vi "IPS120_status.vi"(0 "Address":T1, 1 "error in":errorcluster) -> (2 "Set point":string, 3 "Real Field":string, 4 "Staus":string, 5 "Magnet Failed?":bool, 6 "Arrive":bool, 7 "error out":errorcluster)   [LabVIEW 2012]
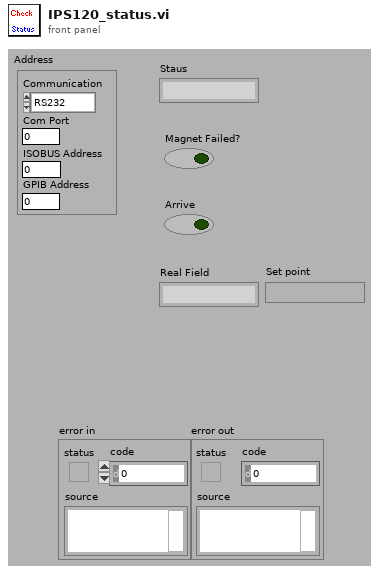
[diagram p1: front panel]
types:
  T1 = cluster{"Com Port":i32, "ISOBUS Address":i32, "GPIB Address":i16, "Communication":enum16{"RS232", "ISOBUS", "GPIB", "Gateway"}}
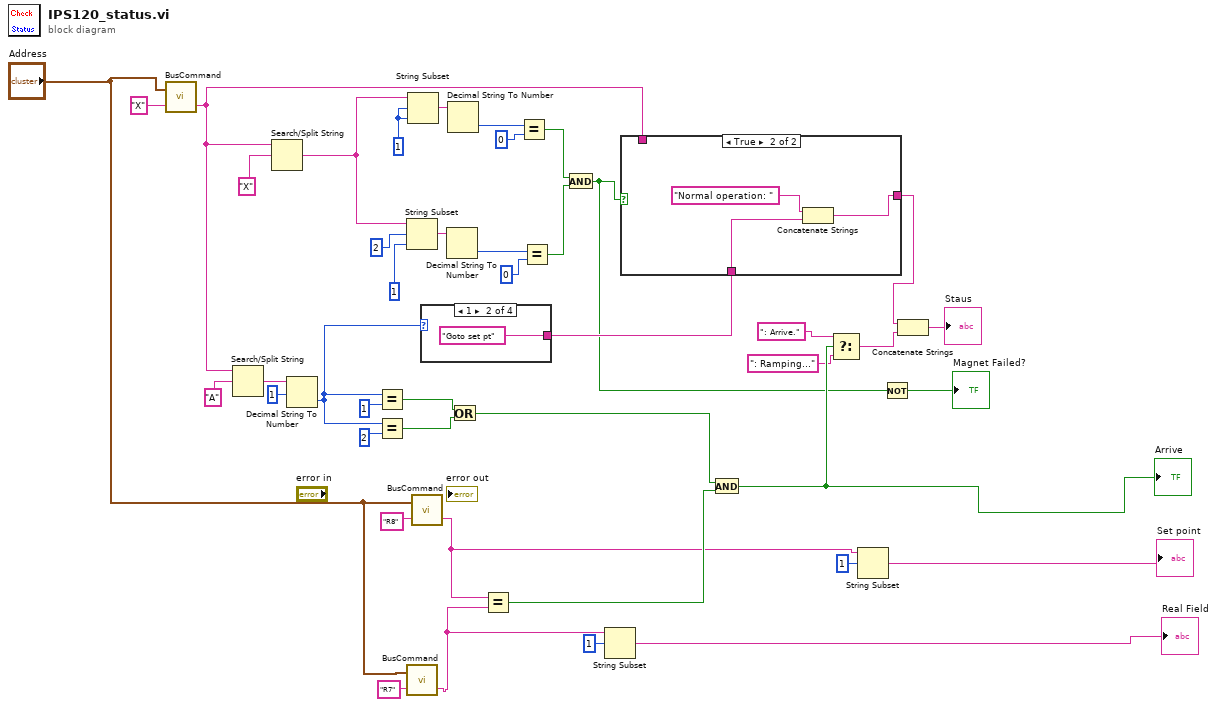
[diagram p0: block diagram]
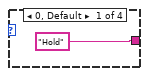
[diagram p2: hidden frame]
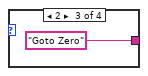
[diagram p3: hidden frame]
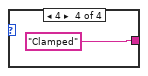
[diagram p4: hidden frame]
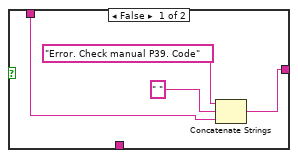
[diagram p5: hidden frame]
diagram:
  w25 = 1
  n1 = call "BusCommand.vi"("Command"="X", "Instrument address (in)"="Address") -> ("Reply"=w7:string)  [unwired: 1 out]
  n2 = Search/Split String(string=w7, search string/char (-)="A") -> (match + rest of string=w21:string)  [unwired: 1 in, 2 out]
  n3 = Search/Split String(string=w7, search string/char (-)="X") -> (match + rest of string=w29:string)  [unwired: 1 in, 2 out]
  n4 = Decimal String To Number(string=w21, offset=1) -> (number=w38:i32)  [unwired: 1 in, 1 out]
  n5 = Equal?(x=w38, y=1) -> (x = y?=w17:bool)
  n6 = Equal?(x=w38, y=2) -> (x = y?=w16:bool)
  n7 = String Subset(string=w29, offset (0)=2, length (rest)=1) -> (substring=w27:string)
  n8 = call "BusCommand.vi"("Command"="R7", "Instrument address (in)"="Address") -> ("Reply"=w4:string)  [unwired: 1 out]
  n9 = String Subset(string=w29, offset (0)=w25, length (rest)=w25) -> (substring=w26:string)
  n10 = call "BusCommand.vi"("Command"="R8", "Instrument address (in)"="Address") -> ("Reply"=w2:string)  [unwired: 1 out]
  n11 = case shown="1" w38 {
    tunnel: ["Hold" "Goto set pt" "Goto Zero" "Clamped"] -> w39
    frame 0, Default {
    }
    frame 1 {
    }
    frame 2 {
    }
    frame 4 {
    }
  }
  n12 = Decimal String To Number(string=w27) -> (number=w34:i32)  [unwired: 2 in, 1 out]
  n13 = Decimal String To Number(string=w26) -> (number=w31:i32)  [unwired: 2 in, 1 out]
  n14 = Or(x=w17, y=w16) -> (x .or. y?=w15:bool)
  n15 = Equal?(x=w2, y=w4) -> (x = y?=w18:bool)
  n16 = Equal?(x=w31, y=0) -> (x = y?=w35:bool)
  n17 = Equal?(x=w34, y=0) -> (x = y?=w36:bool)
  n18 = And(x=w35, y=w36) -> (x .and. y?=w37:bool)
  n19 = String Subset(string=w4, offset (0)=1) -> (substring=→"Real Field":string)  [unwired: 1 in]
  n20 = case shown="True" w37 {
    tunnel: [w50 w52] -> w11
    tunnel: w7 -> [w49 _]
    tunnel: w39 -> [_ w53]
    frame False {
      n21 = Concatenate Strings("Error. Check manual P39. Code", " " ("string"), w49) -> (w50:string)
    }
    frame True {
      n22 = Concatenate Strings("Normal operation: ", w53) -> (w52:string)
    }
  }
  n23 = And(x=w15, y=w18) -> (x .and. y?=w40:bool)
  "Arrive" <- w40
  n24 = Select(t=": Arrive." ("f"), s=w40, f=": Ramping...") -> (s? t:f=w12:string)
  n25 = String Subset(string=w2, offset (0)=1) -> (substring=→"Set point":string)  [unwired: 1 in]
  n26 = Not(x=w37) -> (.not. x?=→"Magnet Failed?":bool)
  n27 = Concatenate Strings(w11, w12) -> (→"Staus":string)
